vi "Camera_Open.vi"(8 "error in":errorcluster, 9 "设备":u16(ring) items=["设备1_22592_3034"], 10 "设备列表":i32[](array[numeric]), 11 "DevCfgGet":cluster{"pid":u32, "vid":u32, "ser_num":u64}[](array[cluster])) -> (0 "error out":errorcluster, 3 "打开设备返回值":i32)   [LabVIEW 2016]
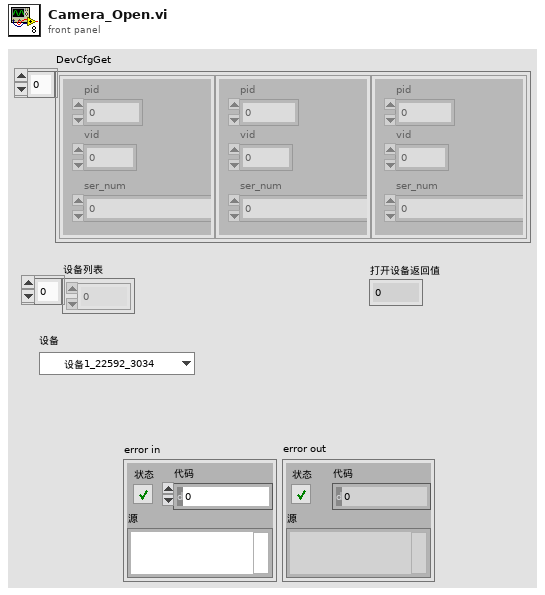
[diagram p1: front panel]
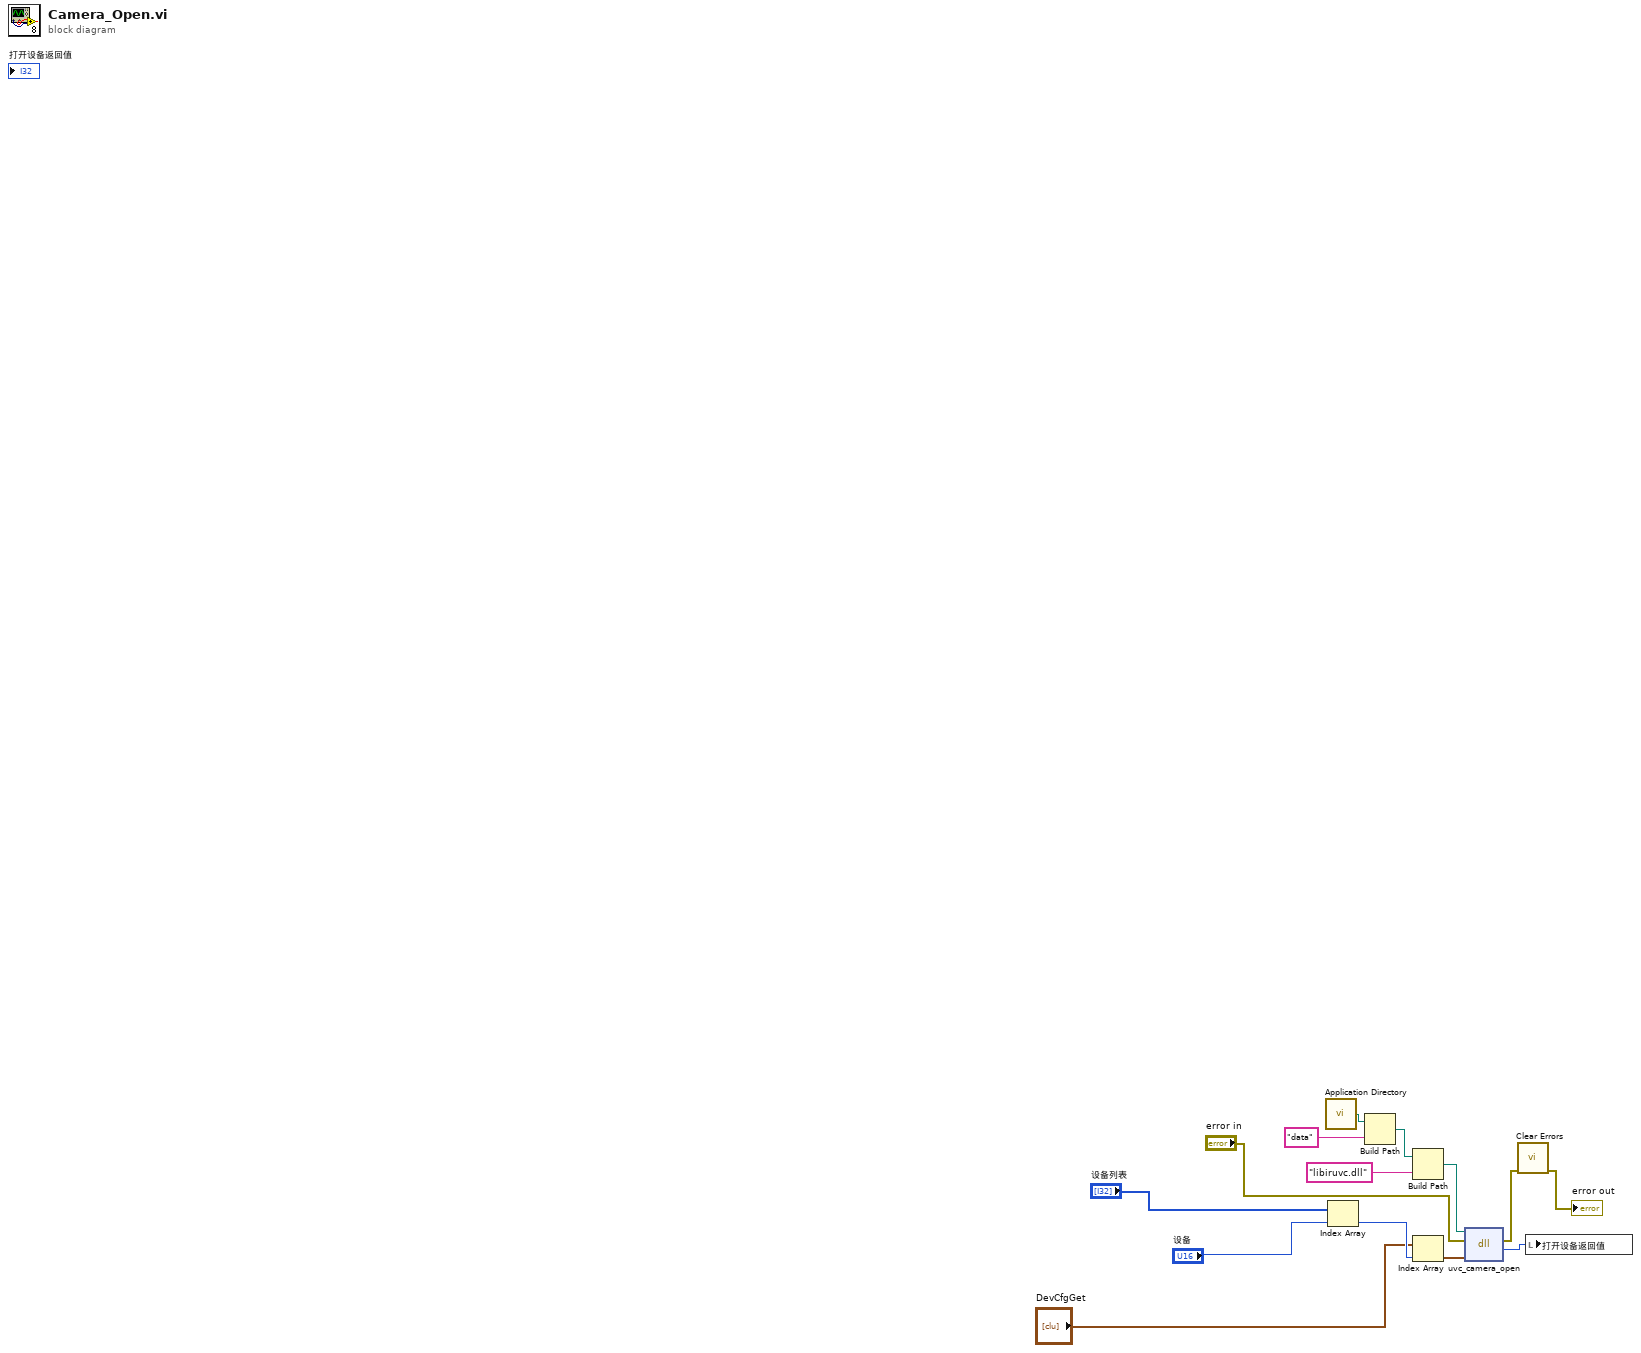
[diagram p0: block diagram]
diagram:
  n1 = call <vilib>:"Application Directory.vi"() -> ("Application Directory"=w12:path)
  n2 = Index Array(array="设备列表", index="设备") -> (element=w7:i32)
  n3 = Build Path(base path=w12, name or relative path="data") -> (appended path=w10:path)
  n4 = Build Path(base path=w10, name or relative path="libiruvc.dll") -> (appended path=w14:path)
  n5 = Index Array(array="DevCfgGet", index=w7) -> (element=w13:cluster{"pid":u32, "vid":u32, "ser_num":u64})
  n6 = dll-call lib="D:/libiruvc_0.3.3/windows/x64/dll/libiruvc.dll" fn="uvc_camera_open"(path in=w14, error in="error in", "dev_cfg"=w13) -> (error out=w2:errorcluster, "return type"=w8:i32)  [unwired: 2 in, 1 out]
  n7 = call <vilib>:"Clear Errors.vi"("error in (no error)"=w2) -> ("error out"=→"error out":errorcluster)  [unwired: 5 in, 1 out]
  n8 = local write "打开设备返回值"(w8) -> ()
